vi "Basic.vi"() -> ()   [LabVIEW 2025]
panel:
  out "Y vs. X":cluster{dbl[], dbl[]}(graph)
  out "T vs. Y position":cluster{dbl[], dbl[]}(graph)
  out "T vs. X position":cluster{dbl[], dbl[]}(graph)
  in  "Initial height (m)":dbl
  in  "Initial speed (m/s)":dbl=1.0 min=1.0
  in  "Angle (degrees)":dbl=1.0 min=1.0 max=89.0
  # "Victor Front Pannel"
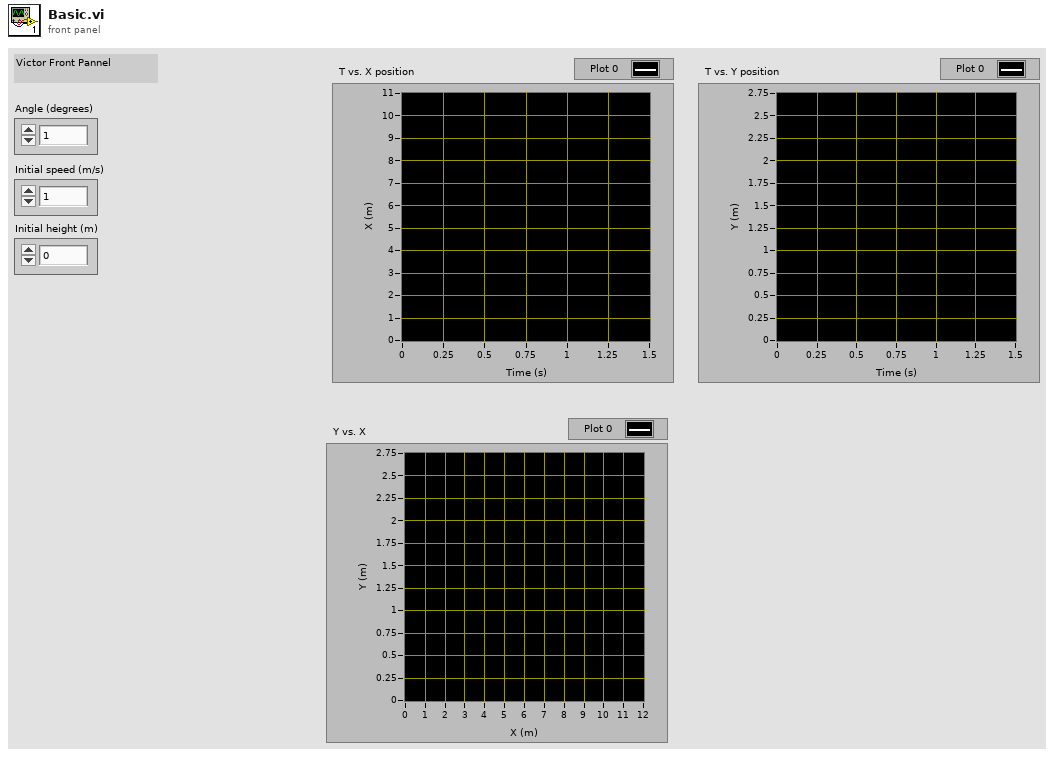
[diagram p1: front panel]
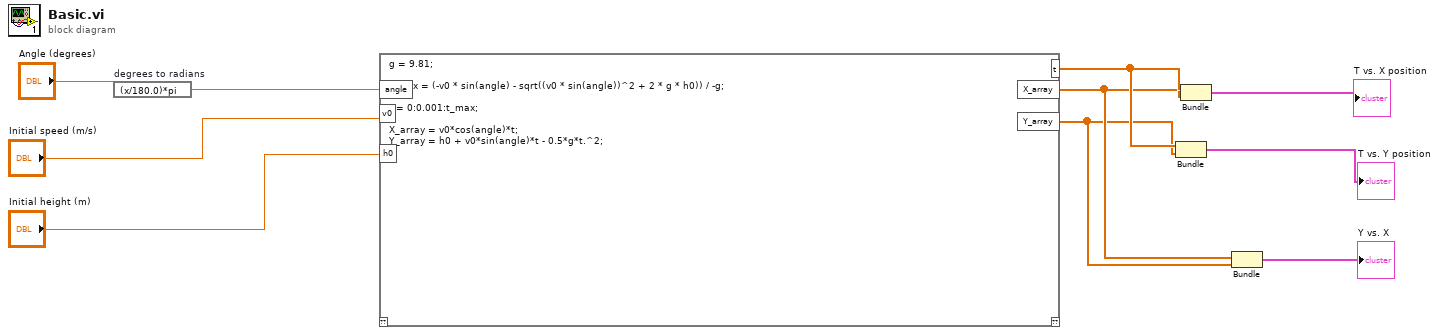
[diagram p0: block diagram]
diagram:
  n1 = expression code="(x/180.0)*pi" "degrees to radians"("Angle (degrees)") -> (w7:dbl)
  n2 = script code="g = 9.81;\n\nt_max = (-v0 * sin(angle) - sqrt((v0 * sin(angle))^2 + 2 * g * h0)) / -g;\n\nt = 0:0.001:t_max;\n\nX_array = v0*cos(angle)*t;\nY_array = h0 + v0*sin(angle)*t - 0.5*g*t.^2;"("angle"=w7, "v0"="Initial speed (m/s)", "h0"="Initial height (m)") -> ("X_array"=w5:dbl[], "Y_array"=w4:dbl[], "t"=w6:dbl[])  [unwired: 1 in, 1 out]
  n3 = Bundle(w6, w4) -> (→"T vs. Y position":cluster{dbl[], dbl[]})  [unwired: 1 in]
  n4 = Bundle(w6, w5) -> (→"T vs. X position":cluster{dbl[], dbl[]})  [unwired: 1 in]
  n5 = Bundle(w5, w4) -> (→"Y vs. X":cluster{dbl[], dbl[]})  [unwired: 1 in]
